vi "Configure Measurement Parameters.vi"(8 "error in (no error)":errorcluster, 9 "Range":dbl=0.02 format="%.2f", 10 "Measurement Function":i32(ring)=10 items=["Continuity", "Current AC", "Current DC", "Diode", "Frequency", "Resistance 4-wire", "Period", "Resistance 2-wire", "Temperature", "Voltage AC", "Voltage DC", "Voltage DC Ratio", "Capacitance"], 11 "VISA resource name":refnum<visa-resource-name>) -> (0 "error out":errorcluster)   [LabVIEW 2015]
uses:
  <instrlib>/Agilent 3446X Series/Agilent 3446X Series.lvlib
panel:
  out "VISA resource name out":refnum<visa-resource-name>
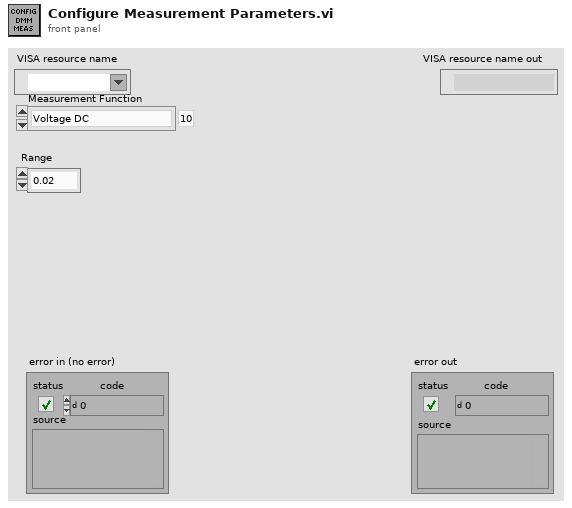
[diagram p1: front panel]
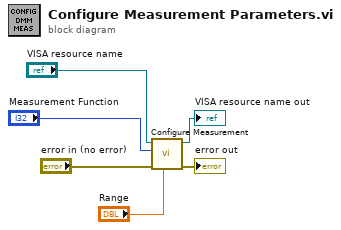
[diagram p0: block diagram]
diagram:
  n1 = call <instrlib>:"Configure Measurement.vi"("Manual Range (1)"="Range", "error in (no error)"="error in (no error)", "Measurement Function (10: Voltage DC)"="Measurement Function", "VISA resource name"="VISA resource name") -> ("error out"=→"error out":errorcluster, "VISA resource name out"=→"VISA resource name out":refnum<visa-resource-name>)  [unwired: 6 in]
